vi "Gaussian fit.vi"(2 "Initial Guess":T1={"Amplitude"=-600.0, "Center"=70.0, "FWHM"=10.0} {"FWHM" format="%.2f"; "Center" format="%.2f"; "Amplitude" format="%.2f"}, 3 "Y":i32[](array[numeric])=[58, 115, 64, 68, 84, 72, 101, 49, 35, 11, 61, 98, 16, 37, 77, 94, 36, 77, 46, 104, 70, 75, 10, 152, 39, 64, 17, 82, 55, 51, 69, 100, 38, 127, 89, 66, 89, 48, 87, 54, 66, 114, 97, 111, 104, 48, 26, 64, 119, 39, 73, 84, 49, -7, 27, 12, 59, 10, 8, 11, 47, 49, 56, 11, -55, -89, -256, -457, -641, -734, -735, -653, -477, -267, -156, -46, -39, 39, -28, 7, -30, 6, 7, 27, 25, 66, 46, 9, 45, 16, 2, 36, 36, 54, -21, 22, 33, -37, 22, 25, 32, -24, 11, 12, 22, 19, 41, 23, 23, 38, 13, -4, -7, 31, 50, 18, 1, 12, -39, 30, 34, 38, -11, 12, 64, 22, -4, -22, -13, -9, 22, -11, 12, -19, -35, -56, 4, -11, 36, 20, 13, 49, -20, 41, 25, 12, 8, -43, -2, 4], 4 "X":dbl[](array[numeric])=[0.0, 1.0, 2.0, 3.0, 4.0, 5.0, 6.0, 7.0, 8.0, 9.0, 10.0, 11.0, 12.0, 13.0, 14.0, 15.0, 16.0, 17.0, 18.0, 19.0, 20.0, 21.0, 22.0, 23.0, 24.0, 25.0, 26.0, 27.0, 28.0, 29.0, 30.0, 31.0, 32.0, 33.0, 34.0, 35.0, 36.0, 37.0, 38.0, 39.0, 40.0, 41.0, 42.0, 43.0, 44.0, 45.0, 46.0, 47.0, 48.0, 49.0, 50.0, 51.0, 52.0, 53.0, 54.0, 55.0, 56.0, 57.0, 58.0, 59.0, 60.0, 61.0, 62.0, 63.0, 64.0, 65.0, 66.0, 67.0, 68.0, 69.0, 70.0, 71.0, 72.0, 73.0, 74.0, 75.0, 76.0, 77.0, 78.0, 79.0, 80.0, 81.0, 82.0, 83.0, 84.0, 85.0, 86.0, 87.0, 88.0, 89.0, 90.0, 91.0, 92.0, 93.0, 94.0, 95.0, 96.0, 97.0, 98.0, 99.0, 100.0, 101.0, 102.0, 103.0, 104.0, 105.0, 106.0, 107.0, 108.0, 109.0, 110.0, 111.0, 112.0, 113.0, 114.0, 115.0, 116.0, 117.0, 118.0, 119.0, 120.0, 121.0, 122.0, 123.0, 124.0, 125.0, 126.0, 127.0, 128.0, 129.0, 130.0, 131.0, 132.0, 133.0, 134.0, 135.0, 136.0, 137.0, 138.0, 139.0, 140.0, 141.0, 142.0, 143.0, 144.0, 145.0, 146.0, 147.0, 148.0, 149.0] format="%.2f") -> (0 "Coefficients":T1 {"FWHM" format="%.2f"; "Center" format="%.2f"; "Amplitude" format="%.2f"}, 1 "Fit":cluster{"X":dbl[], dbl[]}[](graph))   [LabVIEW 2009]
uses:
  <vilib>/gmath/NI_Gmath.lvlib
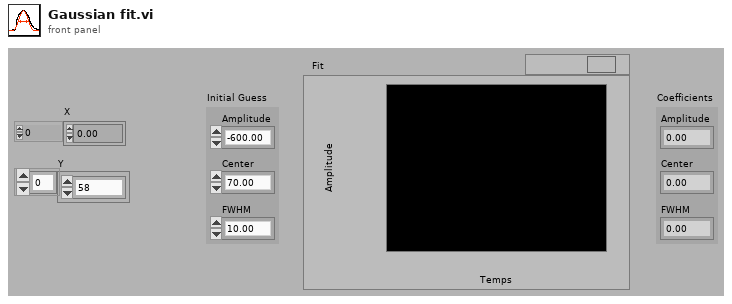
[diagram p1: front panel]
types:
  T1 = cluster{"Amplitude":dbl, "Center":dbl, "FWHM":dbl}
  T2 = cluster{"model":string, "Parameters":string[], "x":string}
  T3 = cluster{"Best Fit Coefficients[0]":dbl, "Best Fit Coefficients[1]":dbl, "Best Fit Coefficients[2]":dbl}
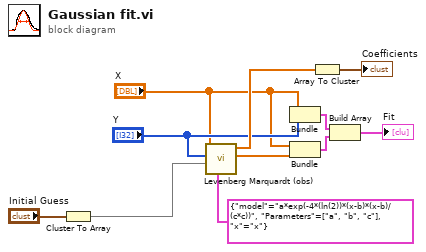
[diagram p0: block diagram]
diagram:
  n1 = Cluster To Array(cluster="Initial Guess") -> (array=w9:dbl[])
  n2 = call <vilib>:"Levenberg Marquardt (obs).vi"("model description"=T2 {"model"="a*exp(-4*(ln(2))*(x-b)*(x-b)/(c*c))", "Parameters"=["a", "b", "c"], "x"="x"}, "Initial Guess Coefficient"=w9, "Y"="Y", "X"="X") -> ("Best Fit"=w4:dbl[], "Best Fit Coefficients"=w7:dbl[])  [unwired: 2 in, 4 out]
  n3 = Bundle("X"="X", "Y"="Y") -> (w2:cluster{"X":dbl[], "Y":i32[]})  [unwired: 1 in]
  n4 = Bundle("X"="X", "Best Fit"=w4) -> (w3:cluster{"X":dbl[], "Best Fit":dbl[]})  [unwired: 1 in]
  n5 = Array To Cluster(array=w7) -> (cluster=→"Coefficients":T3)
  n6 = Build Array(w2, w3) -> (→"Fit":cluster{"X":dbl[], "Best Fit":dbl[]}[])
